vi "MakeUnique1DTable.vi"(11 "Array":string[](array[string])) -> (3 "String":string)   [LabVIEW 2021, in "ButtonBarFlow.lvlib"]
uses:
  ButtonBarFlow.lvlib
  56d25eec-7578-4836-a4ec-97f64050f9a1.vi
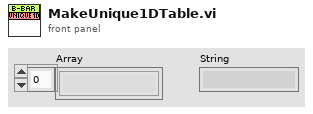
[diagram p1: front panel]
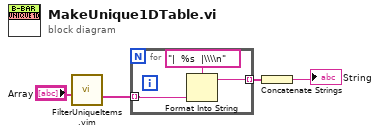
[diagram p0: block diagram]
diagram:
  n1 = call "FilterUniqueItems.vim"("ArrayIn"="Array") -> ("ArrayOut"=w2:string[])  [unwired: 10 in]
  n2 = for {
    tunnel: w2 -> [w7] mode=indexing
    tunnel: [w5] -> w3 mode=indexing
    n3 = Format Into String(format string="|  %s  |\\\\n", w7) -> (resulting string=w5:string)  [unwired: 2 in, 1 out]
  }
  n4 = Concatenate Strings(w3) -> (→"String":string)
